vi "demo-python-postvi.vi"() -> ()   [LabVIEW 2025]
panel:
  in  "Sensors":string
  in  "Operator Name":string
  in  "EnvironmentID":string
  in  "SampleID":string
  out "JSON Response":string
  in  "TestID":string
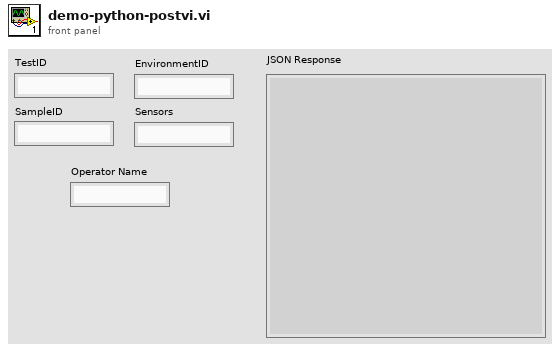
[diagram p1: front panel]
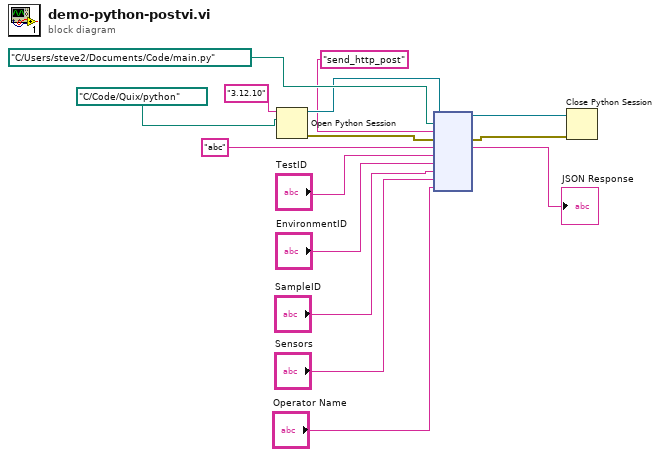
[diagram p0: block diagram]
diagram:
  n1 = Open Python Session(python version="3.12.10", python path=path "C:/Code/Quix/python") -> (session out=w10:refnum<k35>, error out=w11:errorcluster)  [unwired: 1 in]
  n2 = node(w10, path "C:/Users/steve2/Documents/Code/main.py", "send_http_post", w11, "abc", "TestID", "EnvironmentID", "SampleID", "Sensors", "Operator Name") -> (w15:refnum<k35>, w14:errorcluster, →"JSON Response":string)  [unwired: 5 in, 2 out]
  n3 = Close Python Session(session in=w15, error in=w14) -> ()  [unwired: 1 out]
